vi "ClearLineToPrompt.vi"(10 "read buffer":string, 11 "Console In":string) -> (3 "String":string)   [LabVIEW 2017]
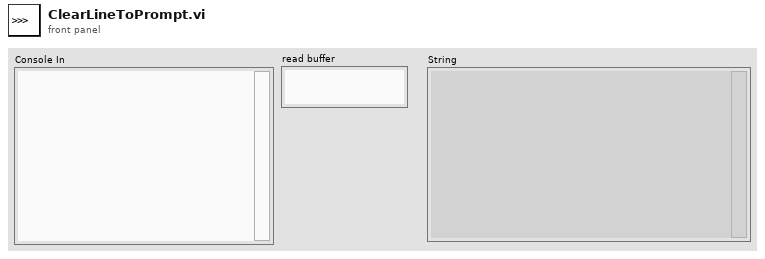
[diagram p1: front panel]
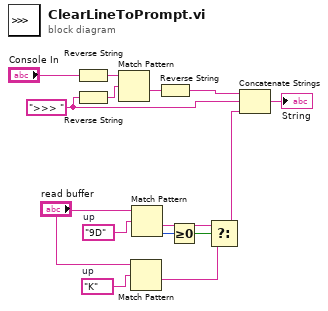
[diagram p0: block diagram]
diagram:
  w7 = "K"  # up
  w8 = "9D"  # up
  w13 = ">>> "
  n1 = Reverse String(1:"Console In") -> (0:w11:string)
  n2 = Reverse String(1:w13) -> (0:w9:string)
  n3 = Match Pattern(string=w11, regular expression=w9) -> (after substring=w10:string)  [unwired: 1 in, 3 out]
  n4 = Match Pattern(string="read buffer", regular expression=w7) -> (after substring=w2:string)  [unwired: 1 in, 3 out]
  n5 = Match Pattern(string="read buffer", regular expression=w8) -> (after substring=w3:string, offset past match=w5:i32)  [unwired: 1 in, 2 out]
  n6 = Reverse String(1:w10) -> (0:w12:string)
  n7 = Greater Or Equal To 0?(x=w5) -> (x >= 0?=w4:bool)
  n8 = Select(t=w3, s=w4, f=w2) -> (s? t:f=w1:string)
  n9 = Concatenate Strings(w12, w13, w1) -> (→"String":string)
